vi "read system hardware ref.vi"(8 "error in":errorcluster, 11 "controller in":refnum<class "Controller.lvclass">) -> (0 "error out":errorcluster, 2 "system hardware ref":refnum<data-value>, 3 "controller out":refnum<class "Controller.lvclass">)   [LabVIEW 2013, in "SMI.lvlib" / "Controller.lvclass"]
uses:
  Controller.lvclass
  Controller.lvclass/Controller.ctl
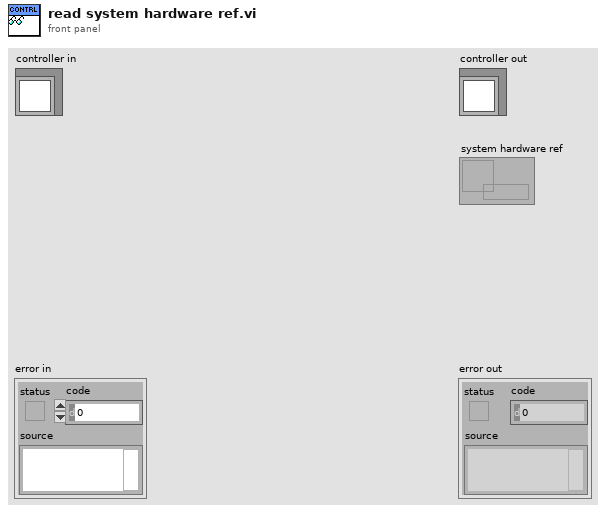
[diagram p1: front panel]
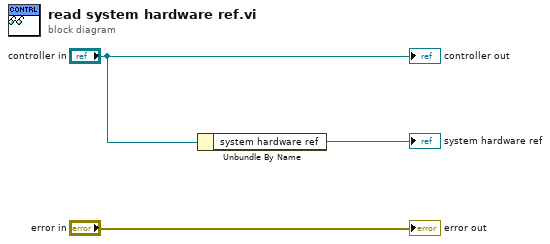
[diagram p0: block diagram]
diagram:
  n1 = Unbundle By Name("controller in") -> ("system hardware ref"=→"system hardware ref":refnum<data-value>)
  "error out" <- "error in"
  "controller out" <- "controller in"
